vi "PQlistAndCreateSequence.vi"(8 "error in":errorcluster, 10 "sequence name":string="serial_n_seq", 11 "conn":u64) -> (0 "error out":errorcluster, 3 "conn_out":u64)   [LabVIEW 2019, in "libpqutility64.lvlib"]
uses:
  libpqutility64.lvlib
  libpqlv64/src/PQresultErrorMessage.vi
  PQclear.vi
  libpqlv64/src/PQsendQuery.vi
  libpqlv64/src/PQgetResult.vi
  libpqlv64/src/PQresultStatus.vi
  PQgetColumn.vi
  libpqlv64/src/PQclear.vi
  PQfetchTables.vi
  libpqlv64/src/PQgetvalue.vi
  libpqlv64/src/PQntuples.vi
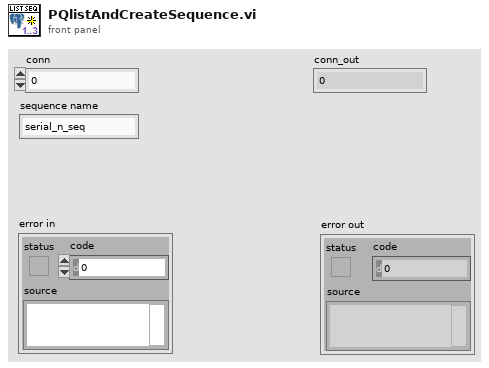
[diagram p1: front panel]
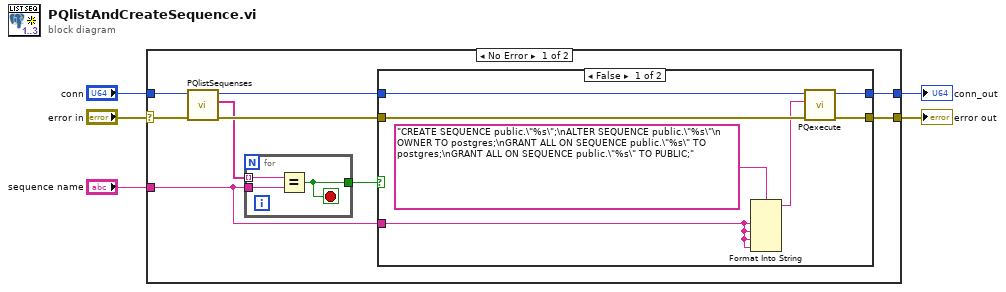
[diagram p0: block diagram]
diagram:
  n1 = case shown="No Error" "error in" {
    selector: "error in" -> [w11 w28]
    tunnel: "conn" -> [w8 w27]
    tunnel: [w14 w27] -> w3
    tunnel: [w13 w28] -> w2
    tunnel: "sequence name" -> [w6 _]
    frame No Error {
      n2 = call "PQlistSequenses.vi"("error in"=w11, "conn"=w8) -> ("error out"=w10:errorcluster, "Data"=w7:string[], "conn_out"=w9:u64)  [unwired: 7 in]
      n3 = for {
        tunnel: w6 -> [w16]
        tunnel: w7 -> [w17] mode=indexing
        tunnel: [w15] -> w12
        stop <- w15 stop-if-true
        n4 = Equal?(x=w17, y=w16) -> (x = y?=w15:bool)
      }
      n5 = case shown="False" w12 {
        tunnel: w9 -> [w24 w26]
        tunnel: [w22 w26] -> w14
        tunnel: w10 -> [w23 w25]
        tunnel: [w21 w25] -> w13
        tunnel: w6 -> [w18 _]
        frame False {
          n6 = Format Into String(format string="CREATE SEQUENCE public.\"%s\";\nALTER SEQUENCE public.\"%s\"\n    OWNER TO postgres;\nGRANT ALL ON SEQUENCE public.\"%s\" TO postgres;\nGRANT ALL ON SEQUENCE public.\"%s\" TO PUBLIC;", w18, w18, w18, w18) -> (resulting string=w19:string)  [unwired: 2 in, 1 out]
          n7 = call "PQexecute.vi"("error in"=w23, "SQL querry"=w19, "conn"=w24) -> ("error out"=w21:errorcluster, "conn_out"=w22:u64)  [unwired: 7 in]
        }
        frame True {
        }
      }
    }
    frame Error {
    }
  }
  "conn_out" <- w3
  "error out" <- w2
